vi "AMI_Desimana Z axis.vi"(6 "error in (no error)":errorcluster, 7 "Index":i8) -> (0 "error out":errorcluster, 3 "resulting string Z":string="Set Magnetic Field 1000.000Tesla at 100.000Tesla/min, Linear, Persistent, Sweep&meas")   [LabVIEW 2017]
doc: "Use this template to create a dialog box. This template polls the state of the buttons on the front panel and does not use events. Use the Dialog Using Events template (not available in Base package) to create a dialog box with event handling."
panel:
  in  "Wait sec":i32=10
  in  "Modo Rampa":u16(ring)=1 items=["RAMP", "PAUSE", "MANUAL UP", "MANUAL DOWN", "ZERO"]
  out "Z Ramp Units":u16(ring)=1 items=["Per SECOND", "Per MINUTE"]
  out "Z Field Units":u16(ring)=1 items=["KGauss", "Tesla"]
  out "Wait stability":bool=TRUE
  in  "Field Mode":i32(ring) items=["Persistent", "Driven"]
  in  "Approach":i32(ring) items=["Linear", "NoOvershoot", "Oscillate"]
  in  "Z rate":dbl=0.03 min=0.0 max=0.1 step=0.001 format="%.2f"
  in  "# steps":i32=1
  out "Cancelled?":bool
  in  "Cancel":bool
  in  "OK":bool
  # "DEMAGNETIZE AXIS Z"
  # "Nov 2022 V2.1  a-sslcdms"
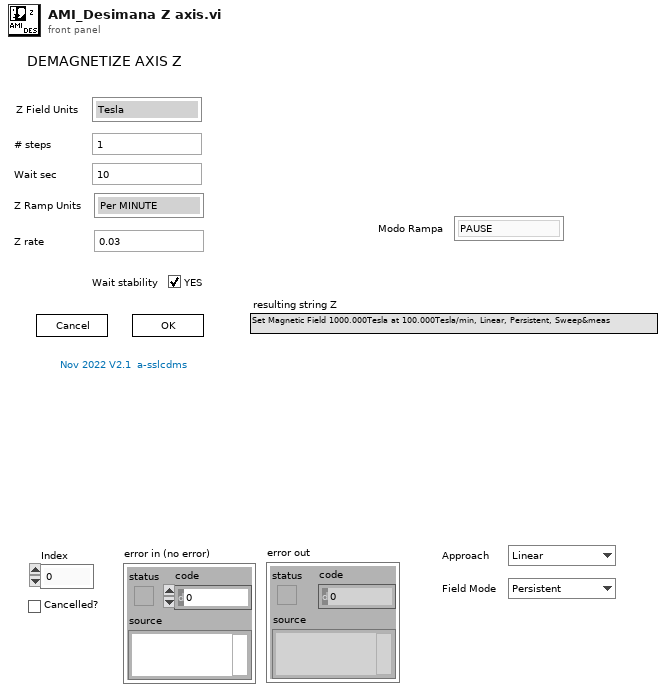
[diagram p1: front panel]
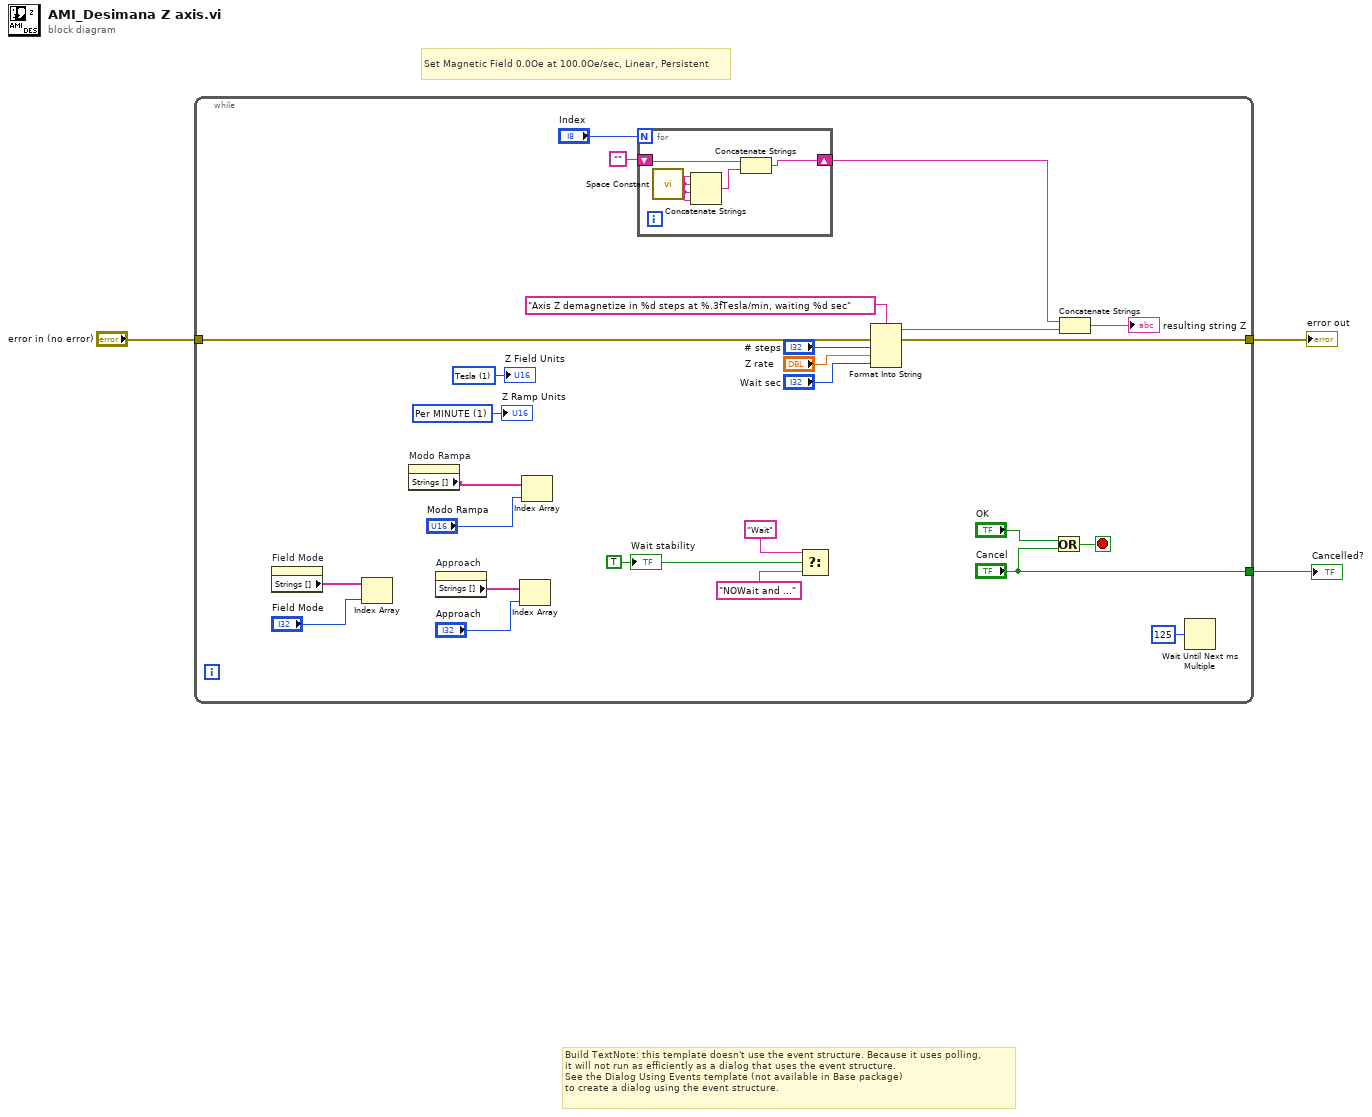
[diagram p0: block diagram]
diagram:
  # "Set Magnetic Field 0.0Oe at 100.0Oe/sec, Linear, Persistent"
  # "Build TextNote: this template doesn't use the event structure. Because it uses polling, \nit will not run as efficiently as a dialog that uses the event structure.\nSee the Dialog Using Events template (not available in Base package) \nto create a dialog using the event structure."
  n1 = while {
    tunnel: ["Cancel"] -> w3
    tunnel: [w7] -> w2
    tunnel: "error in (no error)" -> [w9]
    stop <- w28 stop-if-true
    w10 = u16 1 items=["Per SECOND", "Per MINUTE"] ("Ramp Units")
    w11 = u16 1 items=["KGauss", "Tesla"] ("Field Units")
    w14 = TRUE ("Wait stability")
    n2 = property on="Field Mode" class="Ring (strict)"() -> ("Strings []"=w17:string[])  [unwired: 2 in, 2 out]
    n3 = Index Array(array=w17, index="Field Mode") -> ()  [unwired: 1 out]
    n4 = property on="Modo Rampa" class="Ring (strict)"() -> ("Strings []"=w5:string[])  [unwired: 2 in, 2 out]
    n5 = property on="Approach" class="Ring (strict)"() -> ("Strings []"=w20:string[])  [unwired: 2 in, 2 out]
    n6 = Index Array(array=w20, index="Approach") -> ()  [unwired: 1 out]
    n7 = Index Array(array=w5, index="Modo Rampa") -> ()  [unwired: 1 out]
    n8 = for {
      N: "Index" -> [_]
      shift-right: [w32] -> w8
      shift-left: "" -> [w31]
      n9 = call <vilib>:"Space Constant.vi"() -> ("String"=w30:string)
      n10 = Concatenate Strings(w30, w30, w30, w30) -> (w33:string)
      n11 = Concatenate Strings(w31, w33) -> (w32:string)
    }
    n12 = Select(t="Wait", s=w14, f="NOWait and ...") -> ()  [unwired: 1 out]
    n13 = Format Into String(format string="Axis Z demagnetize in %d steps at %.3fTesla/min, waiting %d sec", error in=w9, "# steps", "Z rate", "Wait sec") -> (resulting string=w22:string, error out=w7:errorcluster)  [unwired: 1 in]
    n14 = Or(x="OK", y="Cancel") -> (x .or. y?=w28:bool)
    n15 = Concatenate Strings(w8, w22) -> (→"resulting string Z":string)
    n16 = Wait Until Next ms Multiple(millisecond multiple=u32 125) -> ()  [unwired: 1 out]
    "Wait stability" <- w14
    "Z Field Units" <- w11
    "Z Ramp Units" <- w10
  }
  "Cancelled?" <- w3
  "error out" <- w2
